vi "Write DAT (1D).vi"(4 "append to file? (new file:F)":bool, 6 "Comments":string, 8 "error in":errorcluster, 9 "Data":dbl[](array[numeric]), 10 "Headers":string[](array[string]), 11 "path":path) -> (0 "error out":errorcluster, 3 "new file path":path)   [LabVIEW 2016, in "Data.DAT.lvclass"]
uses:
  Data.DAT.lvclass
  <vilib>/Utility/file.llb/Write Delimited Spreadsheet (string).vi
panel:
  out "appended array":string[][](array[string])
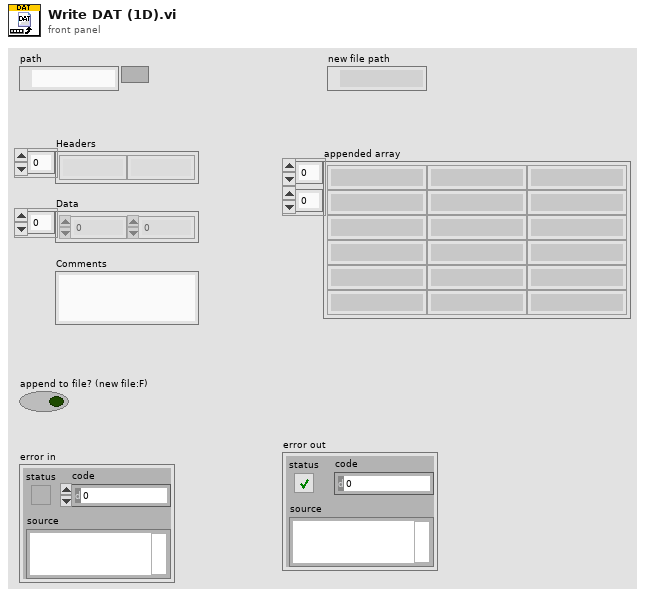
[diagram p1: front panel]
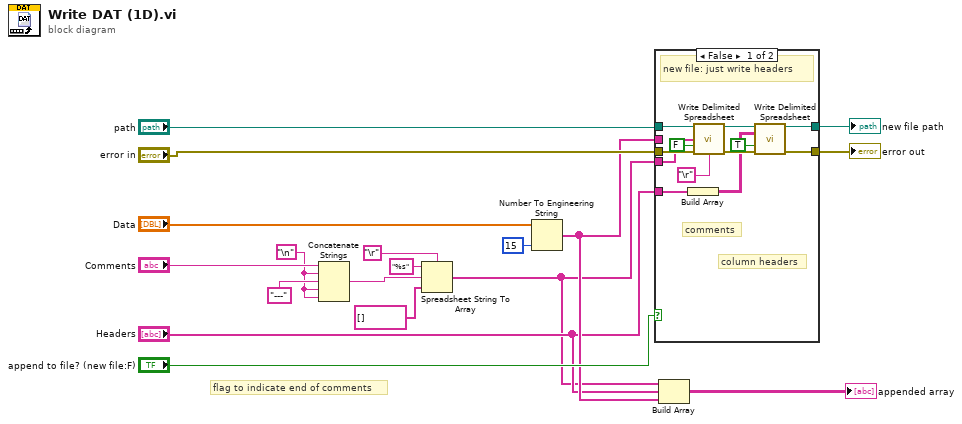
[diagram p0: block diagram]
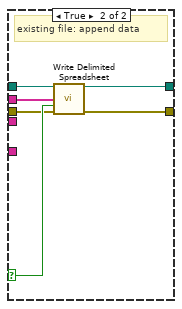
[diagram p2: hidden frame]
diagram:
  w6 = "\n"
  # "flag to indicate end of comments"
  n1 = Concatenate Strings("Comments", w6, "---" ("string"), w6, w6) -> (w11:string)
  n2 = Spreadsheet String To Array(delimiter (Tab)="\r", format string="%s", spreadsheet string=w11, array type (2D Dbl)=string[] []) -> (array=w2:string[])
  n3 = Number To Engineering String(2:i16 15 ("precision (6)"), 4:"Data") -> (0:w4:string[])  [unwired: 2 out]
  n4 = case shown="False" "append to file? (new file:F)" {
    selector: "append to file? (new file:F)" -> [_ w35]
    tunnel: w2 -> [w23 _]
    tunnel: [w28 w32] -> w13
    tunnel: w4 -> [_ w34]
    tunnel: "path" -> [w30 w36]
    tunnel: "error in" -> [w29 w33]
    tunnel: [w25 w31] -> w12
    tunnel: "Headers" -> [w22 _]
    frame False {
      # "column headers"
      # "comments"
      # "new file: just write headers"
      n5 = Build Array(w22) -> (w21:string[][])
      n6 = call-poly <vilib>:"Write Delimited Spreadsheet.vi"("file path (dialog if empty)"=w30, "1D data"=w23, "append to file? (new file:F)"=FALSE, "error in (no error)"=w29, "delimiter (\\t)"="\r") -> ("new file path (Not A Path if cancelled)"=w26:path, "error out"=w27:errorcluster)  [unwired: 9 in]
      n7 = call-poly <vilib>:"Write Delimited Spreadsheet.vi"("file path (dialog if empty)"=w26, "2D data"=w21, "append to file? (new file:F)"=TRUE, "error in (no error)"=w27) -> ("new file path (Not A Path if cancelled)"=w28:path, "error out"=w25:errorcluster)  [unwired: 10 in]
    }
    frame True {
      # "existing file: append data"
      n8 = call-poly <vilib>:"Write Delimited Spreadsheet.vi"("file path (dialog if empty)"=w36, "1D data"=w34, "append to file? (new file:F)"=w35, "error in (no error)"=w33) -> ("new file path (Not A Path if cancelled)"=w32:path, "error out"=w31:errorcluster)  [unwired: 10 in]
    }
  }
  "new file path" <- w13
  "error out" <- w12
  n9 = Build Array(w2, "Headers", w4) -> (→"appended array":string[][])
